vi "W&B Calculator - Deniz Erselcan.vi"() -> ()   [LabVIEW 2026]
panel:
  in  "Remaining Fuel":dbl
  in  "Start Button":bool
  out "Main Check":bool
  in  "Taxi Fuel":dbl
  in  "Stop":bool
  out "Landing Condition Arm Sum":dbl
  out "Landing Condition Mass Sum":dbl
  out "Landing Condition Moment Sum":dbl
  out "Landing Condition Indicator":bool
  out "Trip Fuel Arm Sum":dbl
  out "Trip Fuel Mass Sum":dbl
  out "Trip Fuel Moment Sum":dbl
  out "Trip Fuel Indicator":bool
  out "Take-Off Condition Arm Sum":dbl
  out "Take-Off Condition Mass Sum":dbl
  out "Take-Off Condition Moment Sum":dbl
  out "Take-Off Condition Indicator":bool
  out "Taxi Fuel Arm Sum":dbl
  out "Start/Taxi Fuel Mass Sum":dbl
  out "Taxi Fuel Moment Sum":dbl
  out "Taxi Indicator":bool
  out "Ramp Condition Arm Sum":dbl
  out "Ramp Condition Mass Sum":dbl
  out "Ramp Condition Moment Sum":dbl
  out "Ramp Condition Indicator":bool
  out "Fuel Loaded Arm Sum":dbl
  out "Fuel Loaded Mass Sum":dbl
  out "Fuel Loaded Moment Sum":dbl
  out "Fuel Loaded Indicator":bool
  out "Zero Fuel Arm Sum":dbl
  out "Zero Fuel Mass Sum":dbl
  out "Zero Fuel Moment Sum":dbl
  out "Zero Fuel Condition Indicator":bool
  out "Baggage Arm Sum":dbl
  out "Baggage Mass Sum":dbl
  out "Baggage Moment Sum":dbl
  out "Baggage Indicator":bool
  out "Rear Seat Arm Sum":dbl
  out "Rear Seat Mass Sum":dbl
  out "Rear Seat Moment Sum":dbl
  out "Rear Seat Indicator":bool
  out "Front Seat Arm Sum":dbl
  out "Front Seat Mass Sum":dbl
  out "Front Seat Moment Sum":dbl
  out "Front Seat Indicator":bool
  out "BEW Arm Sum":dbl
  out "BEW Mass Sum":dbl
  out "BEW Moment Sum":dbl
  out "BEW Indicator":bool
  out "Landing CG":dbl caption="CG"
  out "Take-Off CG":dbl caption="CG"
  out "Baggage Weight Check":dbl caption="kg"
  out "Landing Weight check":dbl caption="kg"
  out "Take-Off Weight Check":dbl caption="kg"
  out "Ramp Weight Check":dbl caption="kg"
  out "Landing CG Check":bool
  out "Take-Off CG Check":bool
  out "Baggage Check":bool
  out "Landing Weight Check":bool
  out "Take-Off Check":bool
  out "Ramp Weight Check":bool
  in  "Trip Fuel":dbl
  out "Baggage Indicator Main":bool caption="Baggae Indicator Main"
  in  "Baggage":dbl
  in  "Passenger 2 (Right)":dbl
  in  "Passenger 1 (Left)":dbl
  in  "Co-Pilot Weight":dbl
  in  "Pilot Weight":dbl
  in  "BEW Arm":dbl
  in  "Basic Emty Weight":dbl
  out "Envelope Graph":cluster{dbl[], dbl[]}[](graph)
  # "Flight Crew"
  # "W & B Check"
  # "Aircraft Empty Weight"
  # "Pilot"
  # "Basic Empty Weight"
  # "kg"
  # "kg"
  # "kg"
  # "BEW Arm"
  # "Co-Pilot"
  # "in"
  # "Baggage"
  # "Passengers"
  # "App Control"
  # "Passenger 1 (Left)"
  # "Baggage"
  # "kg"
  # "kg"
  # "kg"
  # "Passenger 2 (Right)"
  # "CG Envelope Graph"
  # "Fuel (Avgas 100LL)"
  # "Loading Summary"
  # "Taxi Fuel"
  # "US Gal"
  # "MTOW"
  # "Trip Fuel"
  # "Basic Empty Weight"
  # "US Gal"
  # "Front Seat (Crew)"
  # "Reserve Fuel"
  # "US Gal"
  # "Rear Seat (Passengers)"
  # "Baggage"
  # "Limit Checks"
  # "Zero Fuel Condition"
  # "Ramp Weight"
  # "Fuel Loaded"
  # "Take-Off Weight"
  # "Ramp Condition"
  # "Landing Weight"
  # "Taxi Fuel"
  # "Baggage Weight"
  # "Take-Off Condition"
  # "Take-Off CG"
  # "Trip Fuel"
  # "Landing CG"
  # "Landing Condition"
  # "● Zero Fuel   ● Ramp   ● Take-Off   ● Landing"
  # "Item                                                     Mass(kg) Arm(in)  Moment   Status"
  # "Beechcraft Bonanza  — Weight & Balance Calculator"
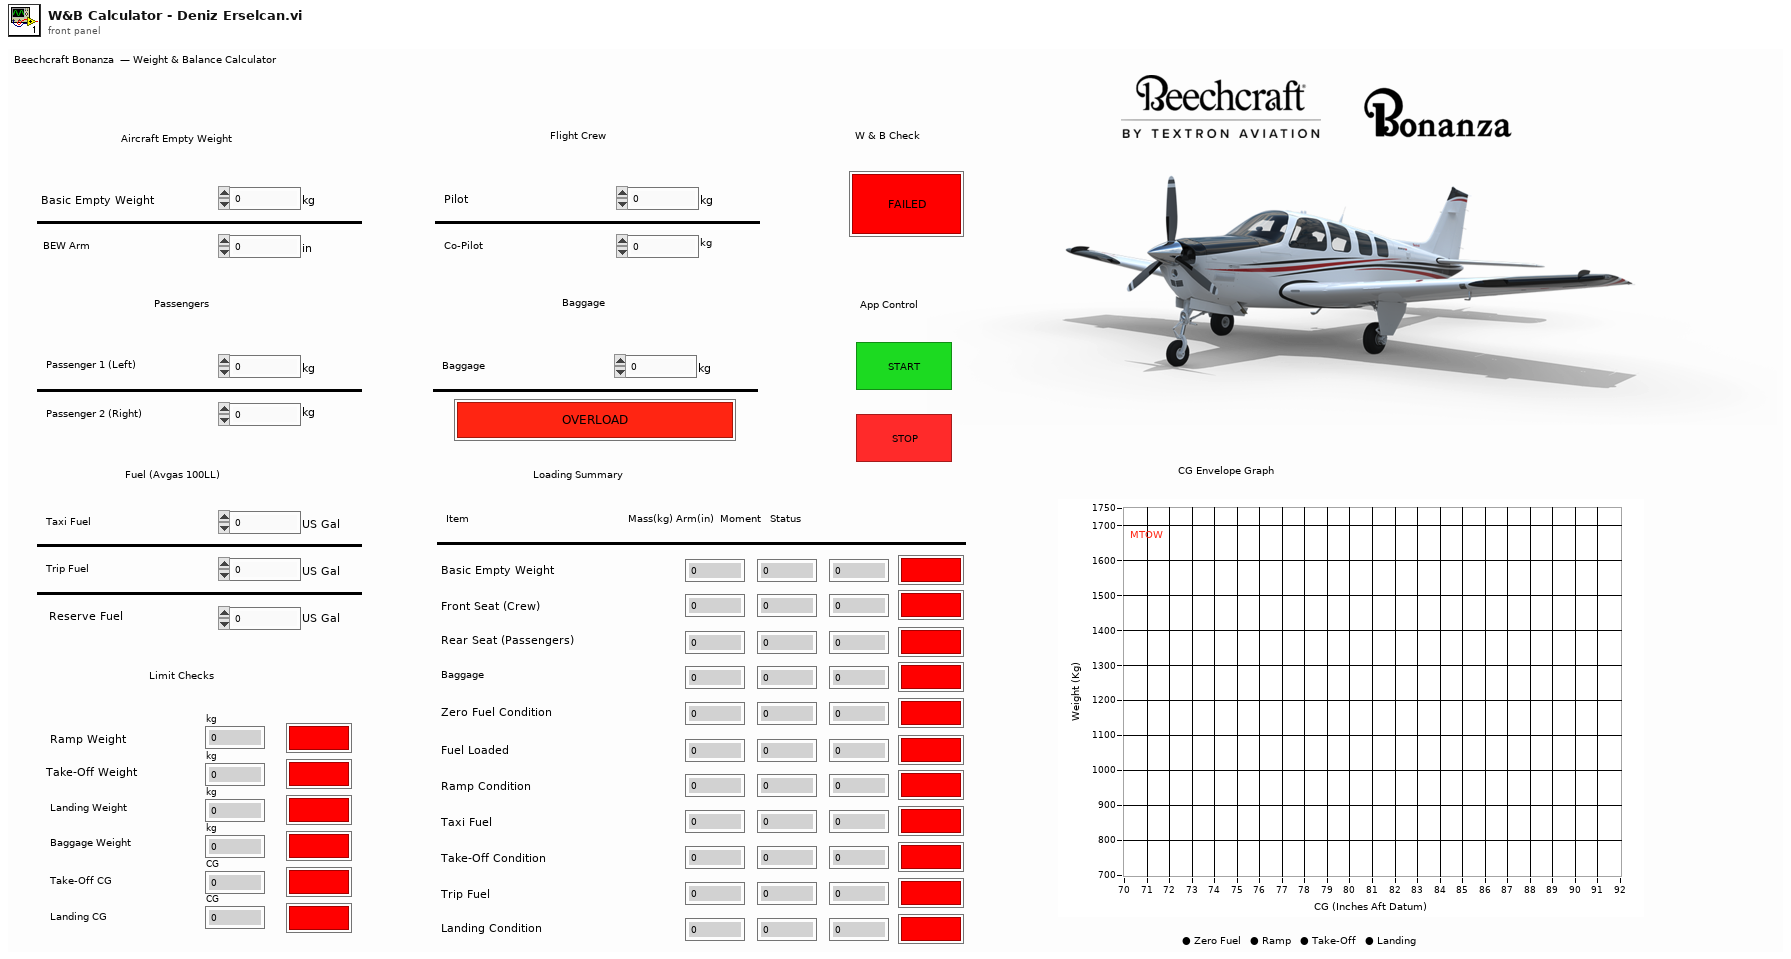
[diagram p1: front panel]
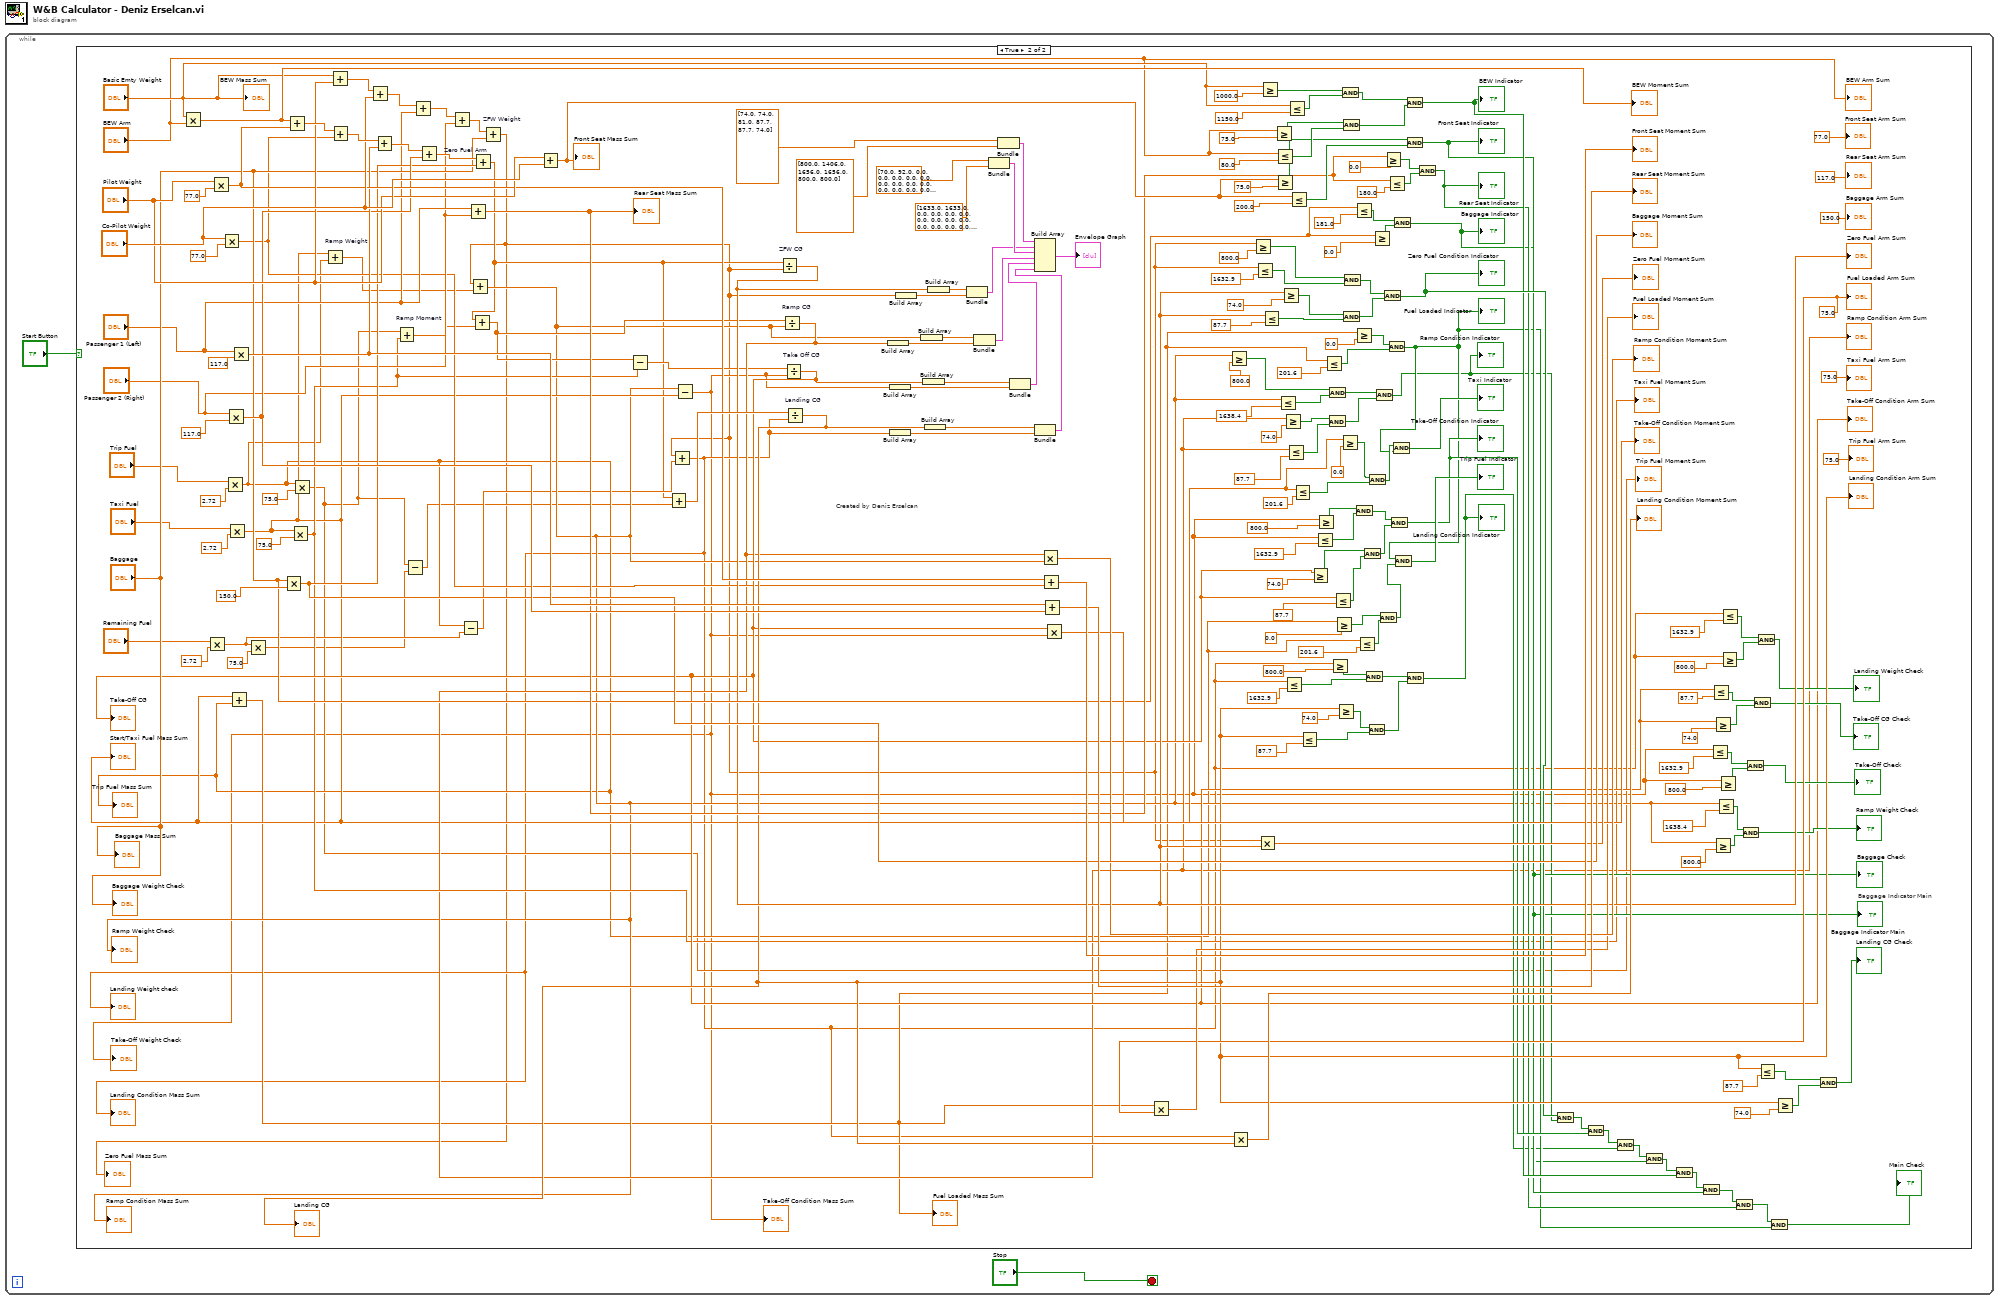
[diagram p0: block diagram]
diagram:
  n1 = while {
    stop <- "Stop" stop-if-true
    n2 = case shown="True" "Start Button" {
      frame False {
      }
      frame True {
        w152 = 75.0
        # "Baggage Indıcator Main"
        # "Created by Deniz Erselcan"
        n3 = Multiply(x="Basic Emty Weight", y="BEW Arm") -> (x*y=w164:dbl)
        "BEW Moment Sum" <- w164
        n4 = Multiply(x="Remaining Fuel", y=2.72) -> (x*y=w12:dbl)
        n5 = Multiply(x="Pilot Weight", y=77.0) -> (x*y=w163:dbl)
        n6 = Multiply(x="Co-Pilot Weight", y=77.0) -> (x*y=w27:dbl)
        n7 = Multiply(x="Trip Fuel", y=2.72) -> (x*y=w13:dbl)
        "Trip Fuel Mass Sum" <- w13
        n8 = Multiply(x="Passenger 2 (Right)", y=117.0) -> (x*y=w160:dbl)
        n9 = Multiply(x="Taxi Fuel", y=2.72) -> (x*y=w22:dbl)
        "Start/Taxi Fuel Mass Sum" <- w22
        n10 = Add(x=w22, y=w13) -> (x+y=w17:dbl)
        "Fuel Loaded Mass Sum" <- w17
        n11 = Multiply(x="Passenger 1 (Left)", y=117.0) -> (x*y=w161:dbl)
        n12 = Multiply(x=w12, y=75.0) -> (x*y=w10:dbl)
        n13 = Multiply(x="Baggage", y=150.0) -> (x*y=w158:dbl)
        "Baggage Moment Sum" <- w158
        n14 = Add(x=w164, y=w163) -> (x+y=w196:dbl)
        n15 = Multiply(x=w22, y=75.0) -> (x*y=w24:dbl)
        "Taxi Fuel Moment Sum" <- w24
        n16 = Multiply(x=w13, y=75.0) -> (x*y=w11:dbl)
        "Trip Fuel Moment Sum" <- w11
        n17 = Add "Ramp Weight"(x=w22, y=w13) -> (x+y=w18:dbl)
        n18 = Add(x="Basic Emty Weight", y="Pilot Weight") -> (x+y=w200:dbl)
        n19 = Add(x=w196, y=w27) -> (x+y=w195:dbl)
        n20 = Add(x=w200, y="Co-Pilot Weight") -> (x+y=w199:dbl)
        n21 = Add(x=w195, y=w161) -> (x+y=w194:dbl)
        n22 = Add "Ramp Moment"(x=w11, y=w24) -> (x+y=w20:dbl)
        n23 = Subtract(x=w11, y=w10) -> (x-y=w5:dbl)
        n24 = Add(x=w199, y="Passenger 1 (Left)") -> (x+y=w198:dbl)
        n25 = Add(x=w194, y=w160) -> (x+y=w193:dbl)
        n26 = Add(x=w198, y="Passenger 2 (Right)") -> (x+y=w197:dbl)
        n27 = Subtract(x=w13, y=w12) -> (x-y=w6:dbl)
        n28 = Add(x="Passenger 1 (Left)", y="Passenger 2 (Right)") -> (x+y=w130:dbl)
        "Rear Seat Mass Sum" <- w130
        n29 = Add "Zero Fuel Arm"(x=w193, y=w158) -> (x+y=w4:dbl)
        n30 = Add(x=w4, y=w20) -> (x+y=w21:dbl)
        n31 = Add "ZFW Weight"(x=w197, y="Baggage") -> (x+y=w3:dbl)
        "Zero Fuel Mass Sum" <- w3
        n32 = Add(x=w3, y=w18) -> (x+y=w19:dbl)
        "Ramp Weight Check" <- w19
        "Ramp Condition Mass Sum" <- w19
        n33 = Add(x="Pilot Weight", y="Co-Pilot Weight") -> (x+y=w135:dbl)
        "Front Seat Mass Sum" <- w135
        n34 = Subtract(x=w21, y=w24) -> (x-y=w7:dbl)
        n35 = Add(x=w4, y=w5) -> (x+y=w181:dbl)
        n36 = Add(x=w3, y=w6) -> (x+y=w9:dbl)
        "Landing Weight check" <- w9
        "Landing Condition Mass Sum" <- w9
        n37 = Subtract(x=w19, y=w22) -> (x-y=w8:dbl)
        "Take-Off Weight Check" <- w8
        "Take-Off Condition Mass Sum" <- w8
        n38 = Divide "ZFW CG"(x=w4, y=w3) -> (x/y=w115:dbl)
        "Zero Fuel Arm Sum" <- w115
        n39 = Divide "Ramp CG"(x=w21, y=w19) -> (x/y=w23:dbl)
        "Ramp Condition Arm Sum" <- w23
        n40 = Divide "Take Off CG"(x=w7, y=w8) -> (x/y=w47:dbl)
        "Take-Off CG" <- w47
        "Take-Off Condition Arm Sum" <- w47
        n41 = Divide "Landing CG"(x=w181, y=w9) -> (x/y=w64:dbl)
        "Landing CG" <- w64
        "Landing Condition Arm Sum" <- w64
        n42 = Build Array(w23) -> (w189:dbl[])
        n43 = Build Array(w8) -> (w182:dbl[])
        n44 = Build Array(w9) -> (w179:dbl[])
        n45 = Build Array(w3) -> (w191:dbl[])
        n46 = Build Array(w19) -> (w188:dbl[])
        n47 = Build Array(w47) -> (w183:dbl[])
        n48 = Build Array(w64) -> (w180:dbl[])
        n49 = Build Array(w115) -> (w192:dbl[])
        n50 = Bundle(w192, w191) -> (w190:cluster{dbl[], dbl[]})  [unwired: 1 in]
        n51 = Bundle(w189, w188) -> (w187:cluster{dbl[], dbl[]})  [unwired: 1 in]
        n52 = Bundle(dbl[] [70.0, 92.0, 0.0, 0.0, 0.0, 0.0, 0.0, 0.0, 0.0, 0.0, 0.0, 0.0, 0.0, 0.0, 0.0, 0.0, 0.0, 0.0, 0.0, 0.0, 0.0, 0.0, 0.0, 0.0, 0.0, 0.0, 0.0, 0.0, 0.0, 0.0, 0.0, 0.0, 0.0, 0.0, 0.0, 0.0, 0.0, 0.0, 0.0, 0.0, 0.0, 0.0, 0.0, 0.0, 0.0, 0.0, 0.0, 0.0, 0.0, 0.0, 0.0, 0.0, 0.0, 0.0, 0.0, 0.0, 0.0, 0.0, 0.0, 0.0, 0.0, 0.0, 0.0, 0.0, 0.0, 0.0, 0.0, 0.0, 0.0, 0.0, 0.0, 0.0, 0.0, 0.0, 0.0, 0.0, 0.0, 77.0], dbl[] [1633.0, 1633.0, 0.0, 0.0, 0.0, 0.0, 0.0, 0.0, 0.0, 0.0, 0.0, 0.0, 0.0, 0.0, 0.0, 0.0, 0.0, 0.0, 0.0, 0.0, 0.0, 0.0, 0.0, 0.0, 0.0, 0.0, 0.0, 0.0, 0.0, 0.0, 0.0, 0.0, 0.0, 0.0, 0.0, 0.0, 0.0, 0.0, 0.0, 0.0, 0.0, 0.0, 0.0, 0.0, 0.0, 0.0, 0.0, 0.0, 0.0, 0.0, 0.0, 0.0, 0.0, 0.0, 0.0, 0.0, 0.0, 0.0, 0.0, 0.0, 0.0, 0.0, 0.0, 0.0, 0.0, 0.0, 0.0, 0.0, 0.0, 0.0, 0.0, 0.0, 0.0, 0.0, 0.0, 0.0, 0.0, 0.0, 0.0, 0.0, 0.0, 0.0, 0.0, 0.0, 0.0, 0.0, 0.0, 0.0, 0.0, 0.0, 0.0, 0.0, 0.0, 0.0, 0.0, 0.0, 0.0, 0.0, 0.0, 0.0, 0.0, 0.0, 0.0, 0.0, 0.0, 0.0, 0.0, 0.0, 0.0, 0.0, 0.0, 0.0, 0.0, 0.0, 0.0, 0.0, 0.0, 0.0, 0.0, 0.0, 0.0, 0.0, 0.0, 0.0, 0.0, 0.0, 0.0, 0.0, 0.0, 0.0, 0.0, 0.0, 0.0, 0.0, 0.0, 0.0, 0.0, 0.0, 0.0, 0.0, 0.0, 0.0, 0.0, 0.0, 0.0, 0.0, 0.0, 0.0, 0.0, 0.0, 0.0, 0.0, 0.0, 0.0, 0.0, 0.0, 0.0, 0.0, 0.0, 0.0, 0.0, 0.0, 0.0, 0.0, 0.0, 0.0, 0.0, 0.0, 0.0, 0.0, 0.0, 0.0, 0.0, 0.0, 0.0, 0.0, 0.0, 0.0, 0.0, 0.0, 0.0, 0.0, 0.0, 0.0, 0.0, 0.0, 0.0, 0.0, 0.0, 0.0, 0.0, 0.0, 0.0, 0.0, 0.0, 0.0, 0.0, 0.0, 0.0, 0.0, 0.0, 0.0, 0.0, 0.0, 0.0, 0.0, 0.0, 0.0, 0.0, 0.0, 0.0, 0.0, 0.0, 0.0, 0.0, 0.0, 0.0, 0.0, 0.0, 0.0, 0.0, 0.0, 0.0, 0.0, 0.0, 0.0, 0.0, 0.0, 0.0, 0.0, 0.0, 0.0, 0.0, 0.0, 0.0, 0.0, 0.0, 0.0, 0.0, 0.0, 0.0, 0.0, 0.0, 0.0, 0.0, 0.0, 0.0, 0.0, 0.0, 0.0, 0.0, 0.0, 0.0, 0.0, 0.0, 0.0, 0.0, 0.0, 0.0, 0.0, 0.0, 0.0, 0.0, 0.0, 0.0, 0.0, 0.0, 0.0, 0.0, 0.0, 0.0, 0.0, 0.0, 0.0, 0.0, 0.0, 0.0, 0.0, 0.0, 0.0, 0.0, 0.0, 0.0, 0.0, 0.0, 0.0, 0.0, 0.0, 0.0, 0.0, 0.0, 0.0, 0.0, 0.0, 0.0, 0.0, 0.0, 0.0, 0.0, 0.0, 0.0, 0.0, 0.0, 0.0, 0.0, 0.0, 0.0, 0.0, 0.0, 0.0, 0.0, 0.0, 0.0, 0.0, 0.0, 0.0, 0.0, 0.0, 0.0, 0.0, 0.0, 0.0, 0.0, 0.0, 0.0, 0.0, 0.0, 0.0, 0.0, 0.0, 0.0, 0.0, 0.0, 0.0, 0.0, 0.0, 0.0, 0.0, 0.0, 0.0, 0.0, 0.0, 0.0, 0.0, 0.0, 0.0, 0.0, 0.0, 0.0, 0.0, 0.0, 0.0, 0.0, 0.0, 0.0, 0.0, 0.0, 0.0, 0.0, 0.0, 0.0, 0.0, 0.0, 0.0, 0.0, 0.0, 0.0, 0.0, 0.0, 0.0, 0.0, 0.0, 0.0, 0.0, 0.0, 0.0, 0.0, 0.0, 0.0, 0.0, 0.0, 0.0, 0.0, 0.0, 0.0, 0.0, 0.0, 0.0, 0.0, 0.0, 0.0, 0.0, 0.0, 0.0, 0.0, 0.0, 0.0, 0.0, 0.0, 0.0, 0.0, 0.0, 0.0, 0.0, 0.0, 0.0, 0.0, 0.0, 0.0, 0.0, 0.0, 0.0, 0.0, 0.0, 0.0, 0.0, 0.0, 0.0, 0.0, 0.0, 0.0, 0.0, 0.0, 0.0, 0.0, 0.0, 0.0, 0.0, 0.0, 0.0, 0.0, 0.0, 0.0, 0.0, 0.0, 0.0, 0.0, 0.0, 0.0, 0.0, 0.0, 0.0, 0.0, 0.0, 0.0, 0.0, 0.0, 0.0, 0.0, 0.0, 0.0, 0.0, 0.0, 0.0, 0.0, 0.0, 0.0, 0.0, 0.0, 0.0, 0.0, 0.0, 0.0, 0.0, 0.0, 0.0, 0.0, 0.0, 0.0, 0.0, 0.0, 0.0, 0.0, 0.0, 0.0, 0.0, 0.0, 0.0, 0.0, 0.0, 0.0, 0.0, 0.0, 0.0, 0.0, 0.0, 0.0, 0.0, 0.0, 0.0, 0.0, 0.0, 0.0, 0.0, 0.0, 0.0, 0.0, 0.0, 0.0, 0.0, 0.0, 0.0, 0.0, 0.0, 0.0, 0.0, 0.0, 0.0, 0.0, 0.0, 0.0, 0.0, 0.0, 0.0, 0.0, 0.0, 0.0, 0.0, 0.0, 0.0, 0.0, 0.0, 0.0, 0.0, 0.0, 0.0, 0.0, 0.0, 0.0, 0.0, 0.0, 0.0, 0.0, 0.0, 0.0, 0.0, 0.0, 0.0, 0.0, 0.0, 0.0, 0.0, 0.0, 0.0, 0.0, 0.0, 0.0, 0.0, 0.0, 0.0, 0.0, 0.0, 0.0, 0.0, 0.0, 0.0, 0.0, 0.0, 0.0, 0.0, 0.0, 0.0, 0.0, 0.0, 0.0, 0.0, 0.0, 0.0, 0.0, 0.0, 0.0, 0.0, 0.0, 0.0, 0.0, 0.0, 0.0, 0.0, 0.0, 0.0, 0.0, 0.0, 0.0, 0.0, 0.0, 0.0, 0.0, 0.0, 0.0, 0.0, 0.0, 0.0, 0.0, 0.0, 0.0, 0.0, 0.0, 0.0, 0.0, 0.0, 0.0, 0.0, 0.0, 0.0, 0.0, 0.0, 0.0, 0.0, 0.0, 0.0, 0.0, 0.0, 0.0, 0.0, 0.0, 0.0, 0.0, 0.0, 0.0, 0.0, 0.0, 0.0, 0.0, 0.0, 0.0, 0.0, 0.0, 0.0, 0.0, 0.0, 0.0, 0.0, 0.0, 0.0, 0.0, 0.0, 0.0, 0.0, 0.0, 0.0, 0.0, 0.0, 0.0, 0.0, 0.0, 0.0, 0.0, 0.0, 0.0, 0.0, 0.0, 0.0, 0.0, 0.0, 0.0, 0.0, 0.0, 0.0, 0.0, 0.0, 0.0, 0.0, 0.0, 0.0, 0.0, 0.0, 0.0, 0.0, 0.0, 0.0, 0.0, 0.0, 0.0, 0.0, 0.0, 0.0, 0.0, 0.0, 0.0, 0.0, 0.0, 0.0, 0.0, 0.0, 0.0, 0.0, 0.0, 0.0, 0.0, 0.0, 0.0, 0.0, 0.0, 0.0, 0.0, 0.0, 0.0, 0.0, 0.0, 0.0, 0.0, 0.0, 0.0, 0.0, 0.0, 0.0, 0.0, 0.0, 0.0, 0.0, 0.0, 0.0, 0.0, 0.0, 0.0, 0.0, 0.0, 0.0, 0.0, 0.0, 0.0, 0.0, 0.0, 0.0, 0.0, 0.0, 0.0, 0.0, 0.0, 0.0, 0.0, 0.0, 0.0, 0.0, 0.0, 0.0, 0.0, 0.0, 0.0, 0.0, 0.0, 0.0, 0.0, 0.0, 0.0, 0.0, 0.0, 0.0, 0.0, 0.0, 0.0, 0.0, 0.0, 0.0, 0.0, 0.0, 0.0, 0.0, 0.0, 0.0, 0.0, 0.0, 0.0, 0.0, 0.0, 0.0, 0.0, 0.0, 0.0, 0.0, 0.0, 0.0, 0.0, 0.0, 0.0, 0.0, 0.0, 0.0, 0.0, 0.0, 0.0, 0.0, 0.0, 0.0, 0.0, 0.0, 0.0, 0.0, 0.0, 0.0, 0.0, 0.0, 0.0, 0.0, 0.0, 0.0, 0.0, 0.0, 0.0, 0.0, 0.0, 0.0, 0.0, 0.0, 0.0, 0.0, 0.0, 0.0, 0.0, 0.0, 0.0, 0.0, 0.0, 0.0, 0.0, 0.0, 0.0, 0.0, 0.0, 0.0, 0.0, 0.0, 0.0, 0.0, 0.0, 0.0, 0.0, 0.0, 0.0, 0.0, 0.0, 0.0, 0.0, 0.0, 0.0, 0.0, 0.0, 0.0, 0.0, 0.0, 0.0, 0.0, 0.0, 0.0, 0.0, 0.0, 0.0, 0.0, 0.0, 0.0, 0.0, 0.0, 0.0, 0.0, 0.0, 0.0, 0.0, 0.0, 0.0, 0.0, 0.0, 0.0, 0.0, 0.0, 0.0, 0.0, 0.0, 0.0, 0.0, 0.0, 0.0, 0.0, 0.0, 0.0, 0.0, 0.0, 0.0, 0.0, 0.0, 0.0, 0.0, 0.0, 0.0, 0.0, 0.0, 0.0, 0.0, 0.0, 0.0, 0.0, 0.0, 0.0, 0.0, 0.0, 0.0, 0.0, 0.0, 0.0, 0.0, 0.0, 0.0, 0.0, 0.0, 0.0, 0.0, 0.0, 0.0, 0.0, 0.0, 0.0, 0.0, 0.0, 0.0, 0.0, 0.0, 0.0, 0.0, 0.0, 0.0, 0.0, 0.0, 0.0, 0.0, 0.0, 0.0, 0.0, 0.0, 0.0, 0.0, 0.0, 0.0, 0.0, 0.0, 0.0, 0.0, 0.0, 0.0, 0.0, 0.0, 0.0, 0.0, 0.0, 0.0, 0.0, 0.0, 0.0, 0.0, 0.0, 0.0, 0.0, 0.0, 0.0, 0.0, 0.0, 0.0, 0.0, 0.0, 0.0, 0.0, 0.0, 0.0, 0.0, 0.0, 0.0, 0.0, 0.0, 0.0, 0.0, 0.0, 0.0, 0.0, 0.0, 0.0, 0.0, 0.0, 0.0, 0.0, 0.0, 0.0, 0.0, 0.0, 0.0, 0.0, 0.0, 0.0, 0.0, 0.0, 0.0, 0.0, 0.0, 0.0, 0.0, 0.0, 0.0, 0.0, 0.0, 0.0, 0.0, 0.0, 0.0, 0.0, 0.0, 0.0, 0.0, 0.0, 0.0, 0.0, 0.0, 0.0, 0.0, 0.0, 0.0, 0.0, 0.0, 0.0, 0.0, 0.0, 0.0, 0.0, 0.0, 0.0, 0.0, 0.0, 0.0, 0.0, 0.0, 0.0, 0.0, 0.0, 0.0, 0.0, 0.0, 0.0, 0.0, 0.0, 0.0, 0.0, 0.0, 0.0, 0.0, 0.0, 0.0, 0.0, 0.0, 0.0, 0.0, 0.0, 0.0, 0.0, 0.0, 0.0, 0.0, 0.0, 0.0, 0.0, 0.0, 0.0, 0.0, 0.0, 0.0, 0.0, 0.0, 0.0, 0.0, 0.0, 0.0, 0.0, 0.0, 0.0, 0.0, 0.0, 0.0, 0.0, 0.0, 0.0, 0.0, 0.0, 0.0, 0.0, 0.0, 0.0, 0.0, 0.0, 0.0, 0.0, 0.0, 0.0, 0.0, 0.0, 0.0, 0.0, 0.0, 0.0, 0.0, 0.0, 0.0, 0.0, 0.0, 0.0, 0.0, 0.0, 0.0, 0.0, 0.0, 0.0, 0.0, 0.0, 0.0, 0.0, 0.0, 0.0, 0.0, 0.0, 0.0, 0.0, 0.0, 0.0, 0.0, 0.0, 0.0, 0.0, 0.0, 0.0, 0.0, 0.0, 0.0, 0.0, 0.0, 0.0, 0.0, 0.0, 0.0, 0.0, 0.0, 0.0, 0.0, 0.0, 0.0, 0.0, 0.0, 0.0, 0.0, 0.0, 0.0, 0.0, 0.0, 0.0, 0.0, 0.0, 0.0, 0.0, 0.0, 0.0, 0.0, 0.0, 0.0, 0.0, 0.0, 0.0, 0.0, 0.0, 0.0, 0.0, 0.0, 0.0, 0.0, 0.0, 0.0, 0.0, 0.0, 0.0, 0.0, 0.0, 0.0, 0.0, 0.0, 0.0, 0.0, 0.0, 0.0, 0.0, 0.0, 0.0, 0.0, 0.0, 0.0, 0.0, 0.0, 0.0, 0.0, 0.0, 0.0, 0.0, 0.0, 0.0, 0.0, 0.0, 0.0, 0.0, 0.0, 0.0, 0.0, 0.0, 0.0, 0.0, 0.0, 0.0, 0.0, 0.0, 0.0, 0.0, 0.0, 0.0, 0.0, 0.0, 0.0, 0.0, 0.0, 0.0, 0.0, 0.0, 0.0, 0.0, 0.0, 0.0, 0.0, 0.0, 0.0, 0.0, 0.0, 0.0, 0.0, 0.0, 0.0, 0.0, 0.0, 0.0, 0.0, 0.0, 0.0, 0.0, 0.0, 0.0, 0.0, 0.0, 0.0, 0.0, 0.0, 0.0, 0.0, 0.0, 0.0, 0.0, 0.0, 0.0, 0.0, 0.0, 0.0, 0.0, 0.0, 0.0, 0.0, 0.0, 0.0, 0.0, 0.0, 0.0, 0.0, 0.0, 0.0, 0.0, 0.0, 0.0, 0.0, 0.0, 0.0, 0.0, 0.0, 0.0, 0.0, 0.0, 0.0, 0.0, 0.0, 0.0, 0.0, 0.0, 0.0, 0.0, 0.0, 0.0, 0.0, 0.0, 0.0, 0.0, 0.0, 0.0, 0.0, 0.0, 0.0, 0.0, 0.0, 0.0, 0.0, 0.0, 0.0, 0.0, 0.0, 0.0, 0.0, 0.0, 0.0, 0.0, 0.0, 0.0, 0.0, 0.0, 0.0, 0.0, 0.0, 1320.0]) -> (w209:cluster{dbl[], dbl[]})  [unwired: 1 in]
        n53 = Bundle(dbl[] [74.0, 74.0, 81.0, 87.7, 87.7, 74.0], dbl[] [800.0, 1406.0, 1656.0, 1656.0, 800.0, 800.0]) -> (w212:cluster{dbl[], dbl[]})  [unwired: 1 in]
        n54 = Bundle(w183, w182) -> (w184:cluster{dbl[], dbl[]})  [unwired: 1 in]
        n55 = Bundle(w180, w179) -> (w178:cluster{dbl[], dbl[]})  [unwired: 1 in]
        n56 = Build Array(w212, w190, w209, w187, w184, w178) -> (→"Envelope Graph":cluster{dbl[], dbl[]}[])
        n57 = Multiply(x=w23, y=w19) -> (x*y=→"Ramp Condition Moment Sum":dbl)
        n58 = Add(x=w163, y=w27) -> (x+y=→"Front Seat Moment Sum":dbl)
        n59 = Add(x=w161, y=w160) -> (x+y=→"Rear Seat Moment Sum":dbl)
        n60 = Multiply(x=w47, y=w8) -> (x*y=→"Take-Off Condition Moment Sum":dbl)
        n61 = Multiply(x=w17, y=w152) -> (x*y=→"Fuel Loaded Moment Sum":dbl)
        n62 = Greater Or Equal?(x=w19, y=800.0) -> (x >= y?=w110:bool)
        n63 = Multiply(x=w9, y=w64) -> (x*y=→"Landing Condition Moment Sum":dbl)
        n64 = Greater Or Equal?(x=w3, y=800.0) -> (x >= y?=w125:bool)
        n65 = Less Or Equal?(x=w3, y=1632.9) -> (x <= y?=w124:bool)
        n66 = Multiply(x=w3, y=w115) -> (x*y=→"Zero Fuel Moment Sum":dbl)
        n67 = Greater Or Equal?(x="Basic Emty Weight", y=1000.0) -> (x >= y?=w149:bool)
        n68 = Less Or Equal?(x=w115, y=87.7) -> (x <= y?=w120:bool)
        n69 = Greater Or Equal?(x="BEW Arm", y=75.0) -> (x >= y?=w144:bool)
        n70 = Less Or Equal?(x="BEW Arm", y=80.0) -> (x <= y?=w140:bool)
        n71 = Greater Or Equal?(x=w135, y=75.0) -> (x >= y?=w139:bool)
        n72 = Less Or Equal?(x=w19, y=1638.4) -> (x <= y?=w109:bool)
        n73 = Greater Or Equal?(x=w115, y=74.0) -> (x >= y?=w121:bool)
        n74 = Greater Or Equal?(x=w23, y=74.0) -> (x >= y?=w106:bool)
        n75 = Less Or Equal?(x=w9, y=1632.9) -> (x <= y?=w81:bool)
        n76 = Less Or Equal?(x=w23, y=87.7) -> (x <= y?=w105:bool)
        n77 = Less Or Equal?(x="Basic Emty Weight", y=1150.0) -> (x <= y?=w148:bool)
        n78 = Less Or Equal?(x=w135, y=200.0) -> (x <= y?=w138:bool)
        n79 = Less Or Equal?(x=w22, y=201.6) -> (x <= y?=w99:bool)
        n80 = Less Or Equal?(x=w64, y=87.7) -> (x <= y?=w77:bool)
        n81 = Greater Or Equal?(x=w47, y=74.0) -> (x >= y?=w92:bool)
        n82 = Less Or Equal?(x=w8, y=1632.9) -> (x <= y?=w95:bool)
        n83 = Greater Or Equal?(x=w8, y=800.0) -> (x >= y?=w96:bool)
        n84 = Less Or Equal?(x=w17, y=201.6) -> (x <= y?=w113:bool)
        n85 = And(x=w106, y=w105) -> (x .and. y?=w101:bool)
        n86 = And(x=w110, y=w109) -> (x .and. y?=w102:bool)
        n87 = Greater Or Equal?(x=w9, y=800.0) -> (x >= y?=w82:bool)
        n88 = Less Or Equal?(x=w47, y=87.7) -> (x <= y?=w91:bool)
        n89 = Greater Or Equal?(x=w13, y=0.0) -> (x >= y?=w86:bool)
        n90 = Greater Or Equal?(x=w64, y=74.0) -> (x >= y?=w78:bool)
        n91 = And(x=w149, y=w148) -> (x .and. y?=w143:bool)
        n92 = Greater Or Equal?(x=w22, y=0.0) -> (x >= y?=w100:bool)
        n93 = And(x=w144, y=w140) -> (x .and. y?=w142:bool)
        n94 = And(x=w121, y=w120) -> (x .and. y?=w116:bool)
        n95 = And(x=w125, y=w124) -> (x .and. y?=w117:bool)
        n96 = Less Or Equal?(x="Baggage", y=181.0) -> (x <= y?=w129:bool)
        n97 = Greater Or Equal?(x=w17, y=0.0) -> (x >= y?=w114:bool)
        n98 = And(x=w96, y=w95) -> (x .and. y?=w88:bool)
        n99 = Less Or Equal?(x=w13, y=201.6) -> (x <= y?=w85:bool)
        n100 = And(x=w92, y=w91) -> (x .and. y?=w87:bool)
        n101 = And(x=w82, y=w81) -> (x .and. y?=w74:bool)
        n102 = And(x=w78, y=w77) -> (x .and. y?=w73:bool)
        n103 = And(x=w100, y=w99) -> (x .and. y?=w71:bool)
        n104 = Greater Or Equal?(x="Baggage", y=0.0) -> (x >= y?=w128:bool)
        n105 = And(x=w102, y=w101) -> (x .and. y?=w30:bool)
        "Ramp Condition Indicator" <- w30
        n106 = And(x=w86, y=w85) -> (x .and. y?=w72:bool)
        n107 = And(x=w117, y=w116) -> (x .and. y?=w43:bool)
        "Zero Fuel Condition Indicator" <- w43
        n108 = Greater Or Equal?(x=w130, y=0.0) -> (x >= y?=w134:bool)
        n109 = Less Or Equal?(x=w130, y=180.0) -> (x <= y?=w133:bool)
        n110 = And(x=w114, y=w113) -> (x .and. y?=w34:bool)
        "Fuel Loaded Indicator" <- w34
        n111 = And(x=w88, y=w87) -> (x .and. y?=w44:bool)
        "Take-Off Condition Indicator" <- w44
        n112 = And(x=w71, y=w34) -> (x .and. y?=→"Taxi Indicator":bool)
        n113 = And(x=w129, y=w128) -> (x .and. y?=w31:bool)
        "Baggage Indicator Main" <- w31
        "Baggage Check" <- w31
        "Baggage Indicator" <- w31
        n114 = And(x=w34, y=w72) -> (x .and. y?=→"Trip Fuel Indicator":bool)
        n115 = And(x=w143, y=w142) -> (x .and. y?=w40:bool)
        "BEW Indicator" <- w40
        n116 = And(x=w139, y=w138) -> (x .and. y?=w38:bool)
        "Front Seat Indicator" <- w38
        n117 = And(x=w74, y=w73) -> (x .and. y?=w29:bool)
        "Landing Condition Indicator" <- w29
        n118 = And(x=w134, y=w133) -> (x .and. y?=w36:bool)
        "Rear Seat Indicator" <- w36
        n119 = And(x=w43, y=w30) -> (x .and. y?=w46:bool)
        n120 = And(x=w46, y=w44) -> (x .and. y?=w45:bool)
        n121 = And(x=w45, y=w29) -> (x .and. y?=w42:bool)
        n122 = And(x=w42, y=w31) -> (x .and. y?=w41:bool)
        n123 = And(x=w41, y=w40) -> (x .and. y?=w39:bool)
        n124 = And(x=w39, y=w38) -> (x .and. y?=w37:bool)
        n125 = Less Or Equal?(x=w8, y=1632.9) -> (x <= y?=w50:bool)
        n126 = Less Or Equal?(x=w47, y=87.7) -> (x <= y?=w68:bool)
        n127 = Greater Or Equal?(x=w47, y=74.0) -> (x >= y?=w67:bool)
        n128 = Greater Or Equal?(x=w19, y=800.0) -> (x >= y?=w55:bool)
        n129 = Less Or Equal?(x=w19, y=1638.4) -> (x <= y?=w54:bool)
        n130 = Greater Or Equal?(x=w8, y=800.0) -> (x >= y?=w51:bool)
        n131 = Greater Or Equal?(x=w9, y=800.0) -> (x >= y?=w59:bool)
        n132 = Less Or Equal?(x=w9, y=1632.9) -> (x <= y?=w58:bool)
        n133 = And(x=w37, y=w36) -> (x .and. y?=w35:bool)
        n134 = And(x=w54, y=w55) -> (x .and. y?=→"Ramp Weight Check":bool)
        n135 = And(x=w50, y=w51) -> (x .and. y?=→"Take-Off Check":bool)
        n136 = And(x=w68, y=w67) -> (x .and. y?=→"Take-Off CG Check":bool)
        n137 = And(x=w58, y=w59) -> (x .and. y?=→"Landing Weight Check":bool)
        n138 = Less Or Equal?(x=w64, y=87.7) -> (x <= y?=w63:bool)
        n139 = And(x=w35, y=w34) -> (x .and. y?=→"Main Check":bool)
        n140 = Greater Or Equal?(x=w64, y=74.0) -> (x >= y?=w62:bool)
        n141 = And(x=w63, y=w62) -> (x .and. y?=→"Landing CG Check":bool)
        "Baggage Weight Check" <- "Baggage"
        "BEW Mass Sum" <- "Basic Emty Weight"
        "BEW Arm Sum" <- "BEW Arm"
        "Front Seat Arm Sum" <- 77.0
        "Rear Seat Arm Sum" <- 117.0
        "Baggage Mass Sum" <- "Baggage"
        "Baggage Arm Sum" <- 150.0
        "Fuel Loaded Arm Sum" <- w152
        "Taxi Fuel Arm Sum" <- 75.0
        "Trip Fuel Arm Sum" <- 75.0
      }
    }
  }
